vi "TDMS_gamepadTwo.vi"(9 "POVs":i16[](array[numeric]), 10 "Buttons":bool[](array[boolean]), 11 "Axes":dbl[](array[numeric])) -> ()   [LabVIEW 2018]
uses:
  <userlib>/836-Library/System/TDMS_V2/Support/TDMS_DevRef.ctl
  <userlib>/836-Library/System/TDMS_V2/Support/Logging_Settings.ctl
  <userlib>/836-Library/System/TDMS_V2/Support/Group_FIFO_Config.ctl
  <userlib>/836-Library/System/TDMS_V2/Support/Channel_FIFO_Config.ctl
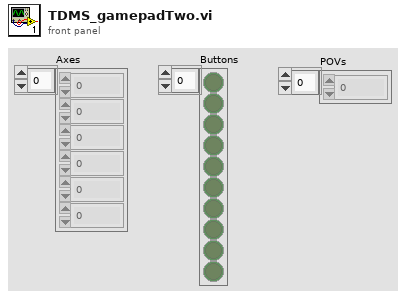
[diagram p1: front panel]
types:
  T1 = typedef "TDMS_DevRef.ctl" = cluster{"Name":string, "File Ref":refnum<k34>, "Start Time":timestamp, "Logging Settings":T2, "Group FIFO Config":T3[], "Data To Write":refnum<data-value>, "semaphore":T5, "Ref Time Reset":refnum<k4>}
  T2 = typedef "Logging_Settings.ctl" = cluster{"Data Grab Period":dbl, "File Write Period":dbl, "Max Stored Size":dbl, "Burst Size":dbl}
  T3 = typedef "Group_FIFO_Config.ctl" = cluster{"Group":string, "Channels":T4[], "Channel Names":string[]}
  T4 = typedef "Channel_FIFO_Config.ctl" = cluster{"Channel":string, "FIFO":refnum<k33>}
  T5 = typedef "Semaphore RefNum" = refnum<k1>
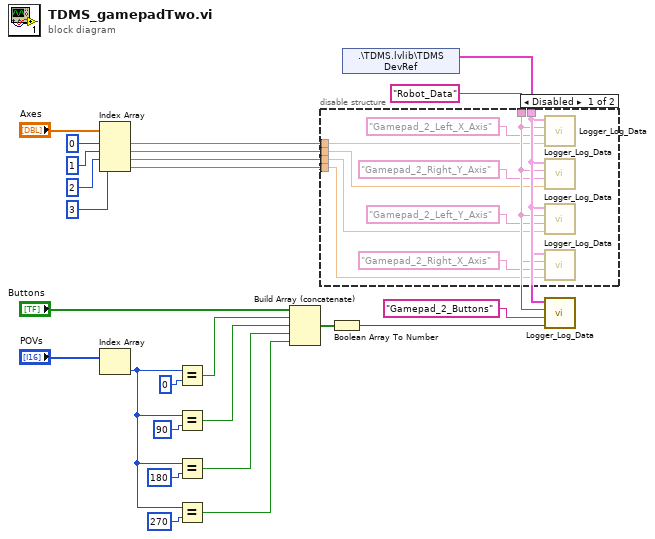
[diagram p0: block diagram]
diagram:
  w16 = "Robot_Data" ("Group")
  n1 = Index Array(array="Axes", index #1=0 ("index"), index #2=1 ("index"), index #3=2 ("index"), index #4=3 ("index")) -> (element #1=w21:dbl, element #2=w19:dbl, element #3=w18:dbl, element #4=w17:dbl)
  n2 = Index Array(array="POVs") -> (element=w10:i16)  [unwired: 1 in]
  n3 = Equal?(x=w10, y=i16 0) -> (x = y?=w6:bool)
  n4 = Equal?(x=w10, y=i16 90) -> (x = y?=w5:bool)
  n5 = Equal?(x=w10, y=i16 180) -> (x = y?=w4:bool)
  n6 = Equal?(x=w10, y=i16 270) -> (x = y?=w3:bool)
  n7 = Build Array (concatenate)("Buttons", w6, w5, w4, w3) -> (w2:bool[])
  n8 = Boolean Array To Number(Boolean array=w2) -> (number=w1:u32)
  n9 = shared-variable ".\\TDMS.lvlib\\TDMS DevRef"() -> (w15:T1)  [unwired: 1 in, 1 out]
  n10 = disable-structure shown="Disabled" {
    disable-tunnel: w21 -> [w31 _]
    disable-tunnel: w19 -> [w30 _]
    disable-tunnel: w18 -> [w29 _]
    disable-tunnel: w17 -> [w28 _]
    disable-tunnel: w16 -> [w27 _]
    disable-tunnel: w15 -> [w26 _]
    frame Disabled {
      n11 = call <userlib>:"Logger_Log_Data.vi"("Data"=w31, "Channel"="Gamepad_2_Left_X_Axis", "Group"=w27, "TDMS DevRef"=w26) -> ()  [unwired: 7 in, 1 out]
      n12 = call <userlib>:"Logger_Log_Data.vi"("Data"=w30, "Channel"="Gamepad_2_Right_Y_Axis", "Group"=w27, "TDMS DevRef"=w26) -> ()  [unwired: 7 in, 1 out]
      n13 = call <userlib>:"Logger_Log_Data.vi"("Data"=w29, "Channel"="Gamepad_2_Left_Y_Axis", "Group"=w27, "TDMS DevRef"=w26) -> ()  [unwired: 7 in, 1 out]
      n14 = call <userlib>:"Logger_Log_Data.vi"("Data"=w28, "Channel"="Gamepad_2_Right_X_Axis", "Group"=w27, "TDMS DevRef"=w26) -> ()  [unwired: 7 in, 1 out]
    }
    frame Enabled {
    }
  }
  n15 = call <userlib>:"Logger_Log_Data.vi"("Data"=w1, "Channel"="Gamepad_2_Buttons", "Group"=w16, "TDMS DevRef"=w15) -> ()  [unwired: 7 in, 1 out]
